vi "GenerateFilePaths.vi"(2 "Logfile?":bool, 3 "DAQmx":bool, 4 "Extension":string=".tdms", 5 "Device Name":string="Sensors_DAQ1") -> (0 "Instrument path":path, 1 "Logfile Path":path=path "C:/Labview Test Data/2018-08-08/Sensors_DAQ1_Log.tdms")   [LabVIEW 2018]
uses:
  Global Variables.vi
  <vilib>/Utility/file.llb/Read Delimited Spreadsheet (string).vi
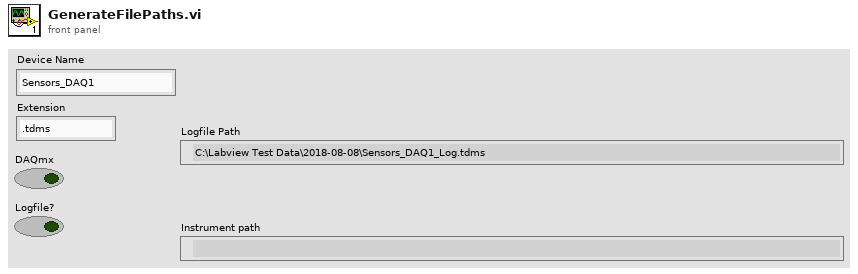
[diagram p1: front panel]
types:
  T1 = cluster{"Project":u16, "SubFolder":string, "Filename (Meas. Description)":string, "Measurement index":i32}
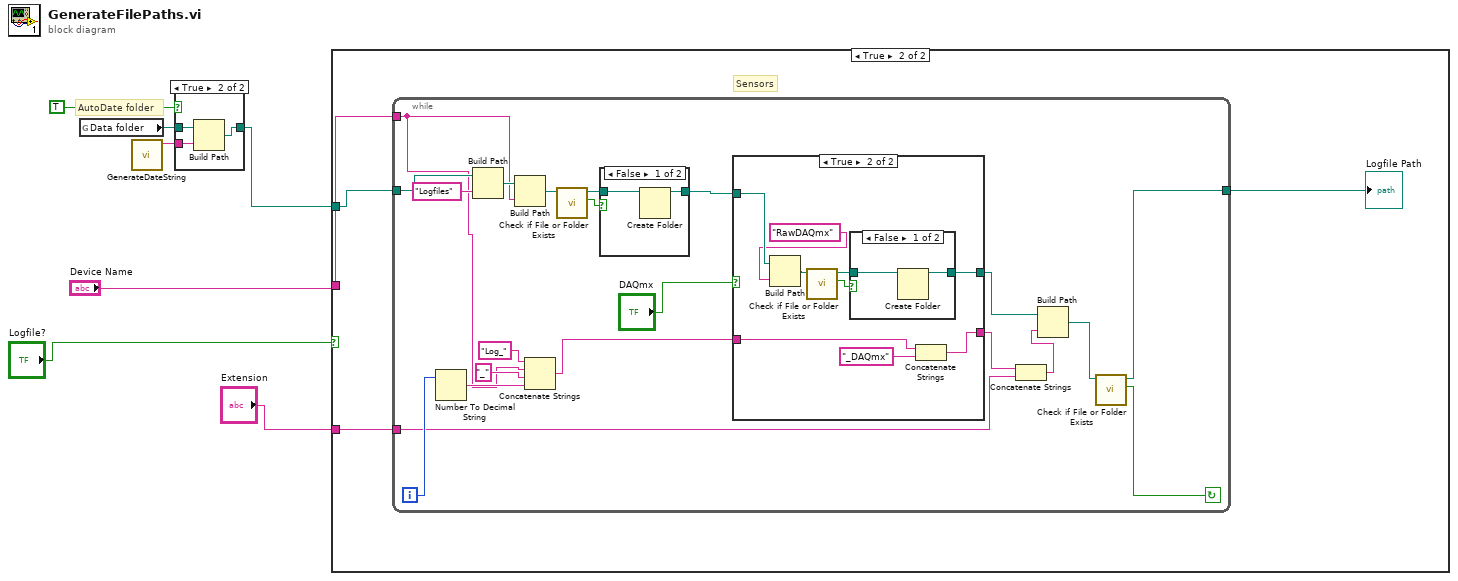
[diagram p0: block diagram]
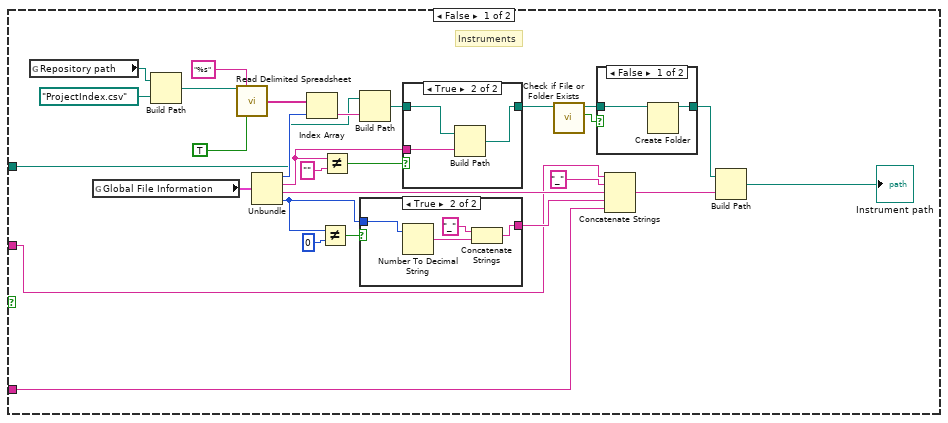
[diagram p2: hidden frame]
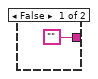
[diagram p5: hidden frame]
diagram:
  # "AutoDate folder"
  n1 = global read "Global Variables.vi" "Data folder"() -> (w5:path)
  n2 = call "GenerateDateString.vi"() -> ("String"=w7:string)  [unwired: 11 in]
  n3 = case shown="True" TRUE ("Auto Date folder") {
    tunnel: w5 -> [w8 w11]
    tunnel: [w8 w9] -> w3
    tunnel: w7 -> [_ w10]
    frame False {
    }
    frame True {
      n4 = Build Path(base path=w11, name or relative path=w10) -> (appended path=w9:path)
    }
  }
  n5 = case shown="True" "Logfile?" {
    tunnel: w3 -> [w14 w54]
    tunnel: "Device Name" -> [w13 w53]
    tunnel: "Extension" -> [w12 w52]
    frame False {
      # "Instruments"
      n6 = global read "Global Variables.vi" "Repository path"() -> (w32:path)
      n7 = global read "Global Variables.vi" "Global File Information"() -> (w37:T1)
      n8 = Build Path(base path=w32, name or relative path=path "ProjectIndex.csv" ("vi path")) -> (appended path=w33:path)
      n9 = call-poly <vilib>:"Read Delimited Spreadsheet.vi"("file path (dialog if empty)"=w33, "format (%s)"="%s", "transpose? (F)"=TRUE) -> ("first row"=w31:string[])  [unwired: 7 in, 5 out]
      n10 = Unbundle(w37) -> ("Project"=w30:u16, "SubFolder"=w19:string, "Filename (Meas. Description)"=w26:string, "Measurement index"=w25:i32)
      n11 = Index Array(array=w31, index=w30) -> (element=w29:string)
      n12 = Not Equal?(x=w25, y=0) -> (x != y?=w38:bool)
      n13 = Not Equal?(x=w19, y="") -> (x != y?=w20:bool)
      n14 = Build Path(base path=w14, name or relative path=w29) -> (appended path=w28:path)
      n15 = case shown="True" w38 {
        tunnel: ["" w50] -> w24
        tunnel: w25 -> [_ w49]
        frame False {
        }
        frame True {
          n16 = Number To Decimal String(number=w49) -> (decimal integer string=w48:string)  [unwired: 1 in]
          n17 = Concatenate Strings("_" ("element"), w48) -> (w50:string)
        }
      }
      n18 = case shown="True" w20 {
        tunnel: w28 -> [w43 w46]
        tunnel: [w43 w45] -> w17
        tunnel: w19 -> [_ w44]
        frame False {
        }
        frame True {
          n19 = Build Path(base path=w46, name or relative path=w44) -> (appended path=w45:path)
        }
      }
      n20 = call <vilib>:"Check if File or Folder Exists.vi"("path"=w17) -> ("file or folder exists?"=w15:bool, "dup path"=w18:path)  [unwired: 8 in, 1 out]
      n21 = case shown="False" w15 {
        tunnel: w18 -> [w41 w42]
        tunnel: [w40 w42] -> w16
        frame False {
          n22 = Create Folder(path (use dialog)=w41) -> (created path=w40:path)  [unwired: 2 in, 2 out]
        }
        frame True {
        }
      }
      n23 = Concatenate Strings(w13, "_" ("string"), w26, w24, w12) -> (w23:string)
      n24 = Build Path(base path=w16, name or relative path=w23) -> (appended path=→"Instrument path":path)
    }
    frame True {
      # "Sensors"
      n25 = while {
        tunnel: w53 -> [w64]
        tunnel: w52 -> [w59]
        tunnel: w54 -> [w65]
        tunnel: [w56] -> w55
        i -> [w61]
        stop <- w62 continue-if-true
        n26 = Number To Decimal String(number=w61) -> (decimal integer string=w69:string)  [unwired: 1 in]
        n27 = Build Path(base path=w65, name or relative path="Logfiles") -> (appended path=w76:path)
        n28 = Build Path(base path=w76, name or relative path=w64) -> (appended path=w71:path)
        n29 = Concatenate Strings("Log_" ("string"), w64, "_" ("string"), w69) -> (w75:string)
        n30 = call <vilib>:"Check if File or Folder Exists.vi"("path"=w71) -> ("file or folder exists?"=w72:bool, "dup path"=w70:path)  [unwired: 8 in, 1 out]
        n31 = case shown="False" w72 {
          tunnel: w70 -> [w92 w93]
          tunnel: [w91 w93] -> w73
          frame False {
            n32 = Create Folder(path (use dialog)=w92) -> (created path=w91:path)  [unwired: 2 in, 2 out]
          }
          frame True {
          }
        }
        n33 = case shown="True" "DAQmx" {
          tunnel: [w77 w86] -> w58
          tunnel: w75 -> [w77 w85]
          tunnel: [w78 w84] -> w74
          tunnel: w73 -> [w78 w81]
          frame False {
          }
          frame True {
            n34 = Build Path(base path=w81, name or relative path="RawDAQmx") -> (appended path=w82:path)
            n35 = call <vilib>:"Check if File or Folder Exists.vi"("path"=w82) -> ("file or folder exists?"=w87:bool, "dup path"=w83:path)  [unwired: 8 in, 1 out]
            n36 = case shown="False" w87 {
              tunnel: w83 -> [w89 w90]
              tunnel: [w88 w90] -> w84
              frame False {
                n37 = Create Folder(path (use dialog)=w89) -> (created path=w88:path)  [unwired: 2 in, 2 out]
              }
              frame True {
              }
            }
            n38 = Concatenate Strings(w85, "_DAQmx" ("string")) -> (w86:string)
          }
        }
        n39 = Concatenate Strings(w58, w59) -> (w57:string)
        n40 = Build Path(base path=w74, name or relative path=w57) -> (appended path=w63:path)
        n41 = call <vilib>:"Check if File or Folder Exists.vi"("path"=w63) -> ("file or folder exists?"=w62:bool, "dup path"=w56:path)  [unwired: 8 in, 1 out]
      }
      "Logfile Path" <- w55
    }
  }
